vi "Request Events.vi"(8 "error in (no error)":errorcluster, 10 "Promise":refnum<class "Promise.lvclass">, 11 "EventHandler in":refnum<class "EventHandler.lvclass">) -> (0 "error out":errorcluster, 3 "EventHandler out":refnum<class "EventHandler.lvclass">)   [LabVIEW 2020, in "Volatus.lvlib" / "EventHandler.lvclass"]
uses:
  EventHandler.lvclass
  lv-promises/Promises/Promise/Promise.lvclass
  EventsValue/EventsValue.lvclass
  C:/dev/lv20CE/relink/lv-promises/Promises/Value/Value.lvclass
  C:/dev/lv20CE/relink/lv-volatus/Volatus/EventsValue/EventsValue.lvclass
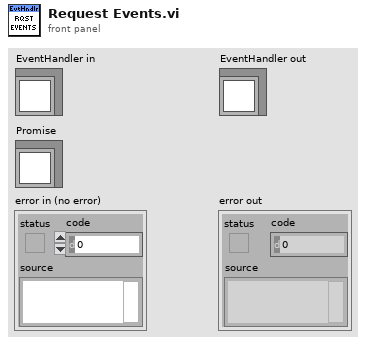
[diagram p1: front panel]
types:
  T1 = typedef "Volatus.lvlib/Event.ctl" = cluster{"Level":T2, "Context":string, "Message":string, "Error":errorcluster}
  T2 = typedef "Volatus.lvlib/Event Level.ctl" = enum16{"Debug", "Info", "Warning", "Error"}
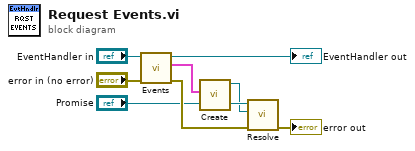
[diagram p0: block diagram]
diagram:
  n1 = call-dynamic "Events.vi"("error in (no error)"="error in (no error)", "EventHandler in"="EventHandler in") -> ("error out"=w8:errorcluster, "Events"=w4:T1[], "EventHandler out"=→"EventHandler out":refnum<class "EventHandler.lvclass">)  [unwired: 7 in]
  n2 = call "Create.vi"("Events"=w4) -> ("EventsValue out"=w2:refnum<class "EventsValue.lvclass">)  [unwired: 10 in]
  n3 = call "Resolve.vi"("error in (no error)"=w8, "Result"=w2, "Promise in"="Promise") -> ("error out"=→"error out":errorcluster)  [unwired: 7 in, 1 out]
